vi "Emballage affiche lot à scanner.vi"(0 "Tableau \nlots OUT":string[][](array[string]), 1 "Affiche ?":bool, 2 "Indice n° lot à scanner":u64, 3 "error in (no error)":errorcluster caption="entrée d'erreur (pas d'erreur)") -> (5 "n° lot à scanner":string, 6 "quantité à scanner de ce lot":i32, 7 "error out":errorcluster caption="sortie d'erreur")   [LabVIEW 2020]
uses:
  Modules/FS/60_FS_Controles/60_FS_SetGet.ctl
panel:
  in  "Bouton confimer":bool
  # "Scanner les valves \ndu lot n°0000"
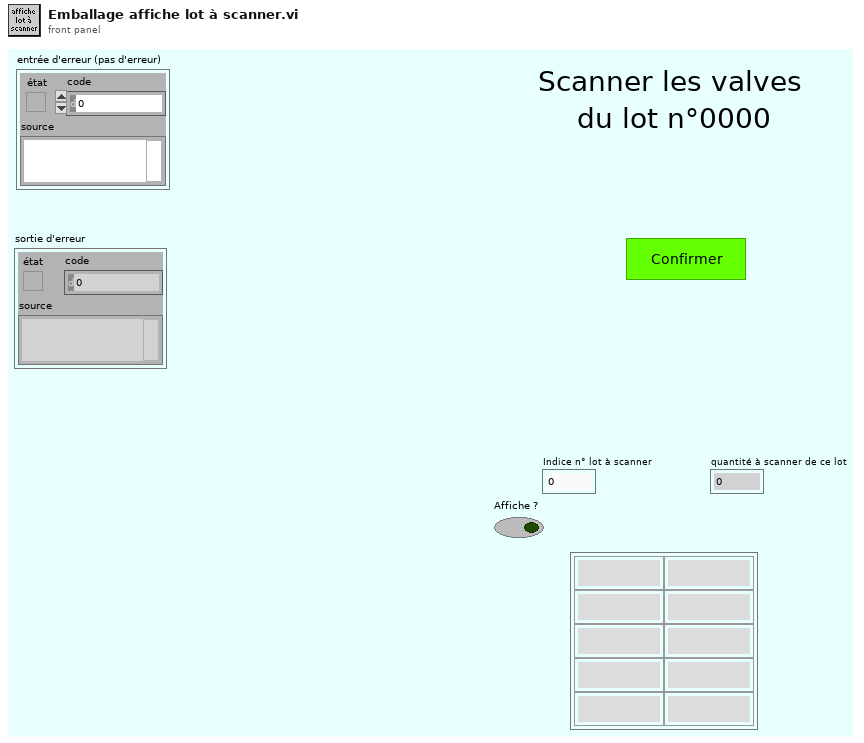
[diagram p1: front panel]
types:
  T1 = typedef "60_FS_SetGet.ctl" = enum16{"set", "get"}
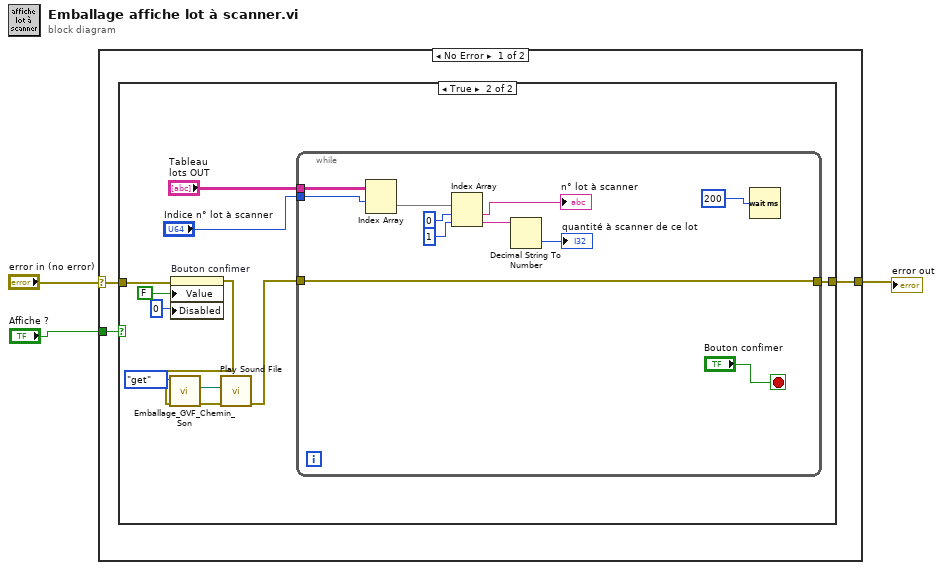
[diagram p0: block diagram]
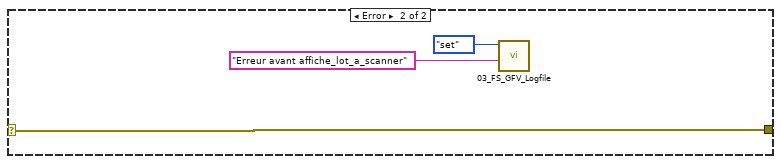
[diagram p3: hidden frame]
diagram:
  n1 = case shown="No Error" "error in (no error)" {
    selector: "error in (no error)" -> [w5 w32]
    tunnel: [w6 w32] -> w2
    tunnel: "Affiche ?" -> [w4 _]
    frame No Error {
      n2 = case shown="True" w4 {
        tunnel: [w7 w18] -> w6
        tunnel: w5 -> [w7 w16]
        frame False {
        }
        frame True {
          n3 = property on="Bouton confimer" class="Bool (strict)"(error in=w16, "Value"=FALSE ("Bouton confimer"), "Disabled"=0) -> (error out=w11:errorcluster)  [unwired: 1 in, 1 out]
          n4 = call "Emballage_GVF_Chemin_Son.vi"("entrée d'erreur (pas d'erreur)"=w11, "Énum"=enum16{"get", "set"}."get") -> ("sortie d'erreur"=w10:errorcluster, "Chemin Utopia - Question.WAV"=w9:path)  [unwired: 5 in, 3 out]
          n5 = call <vilib>:"Play Sound File.vi"("error in (no error)"=w10, "path"=w9) -> ("error out"=w12:errorcluster)  [unwired: 8 in, 1 out]
          n6 = while {
            tunnel: w12 -> [w29]
            tunnel: [w29] -> w18
            tunnel: "Tableau \nlots OUT" -> [w26]
            tunnel: "Indice n° lot à scanner" -> [w25]
            stop <- "Bouton confimer" stop-if-true
            n7 = Index Array(array=w26, index (row)=w25) -> (element=w24:string[])  [unwired: 1 in]
            n8 = Index Array(array=w24, index #1=0, index #2=1) -> (element #1=→"n° lot à scanner":string, element #2=w20:string)
            n9 = Decimal String To Number(string=w20) -> (number=→"quantité à scanner de ce lot":i32)  [unwired: 2 in, 1 out]
            n10 = Wait (ms)(milliseconds to wait=u32 200 ("valeur de l'horloge en ms")) -> ()  [unwired: 1 out]
          }
        }
      }
    }
    frame Error {
      n11 = call "03_FS_GFV_Logfile.vi"("Chaîne"="Erreur avant affiche_lot_a_scanner", "States"=60_FS_SetGet."set") -> ()  [unwired: 8 in, 2 out]
    }
  }
  "error out" <- w2
